vi "Start Fan.vi"(8 "error in (no error)":errorcluster, 10 "Fan Speed":dbl, 11 "iFan Controller in":refnum<class "iFan Controller.lvclass">) -> (0 "error out":errorcluster, 3 "iFan Controller out":refnum<class "iFan Controller.lvclass">)   [LabVIEW 2019, in "iFan Controller.lvclass"]
uses:
  <vilib>/gpm_packages/@cs/Car-wash/Source/iFan Controller/iFan Controller.lvclass
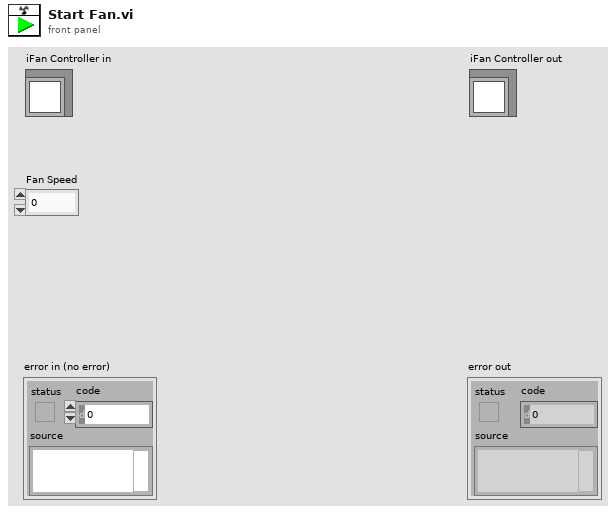
[diagram p1: front panel]
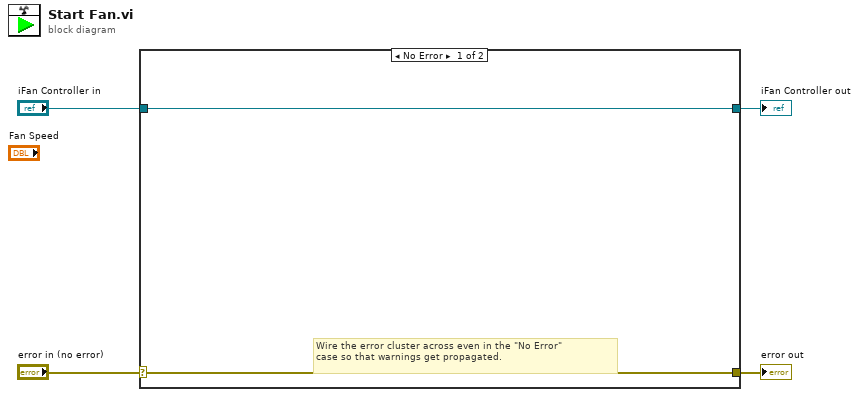
[diagram p0: block diagram]
diagram:
  n1 = case shown="No Error" "error in (no error)" {
    selector: "error in (no error)" -> [w5 w8]
    tunnel: [w5 w8] -> w3
    tunnel: [w6 w7] -> w1
    tunnel: "iFan Controller in" -> [w6 w7]
    frame No Error {
      # "Wire the error cluster across even in the \"No Error\"\ncase so that warnings get propagated."
    }
    frame Error {
    }
  }
  "error out" <- w3
  "iFan Controller out" <- w1
